vi "Calculate Image MSE.vi"(8 "error in (no error)":errorcluster, 10 "Actual Image":T1, 11 "Expected Image":T1) -> (0 "error out":errorcluster, 3 "MSE":dbl)   [LabVIEW 2020, in "MacroAssert.lvlib" / "Image Assertion.lvclass"]
doc: "Calculates the mean squared error (MSE) between <B>Expected Image</B> and <B>Actual Image</B>."
uses:
  Image Assertion.lvclass
  <vilib>/picture/picture.llb/imagedata.ctl
  <vilib>/Analysis/NI_AALPro.lvlib
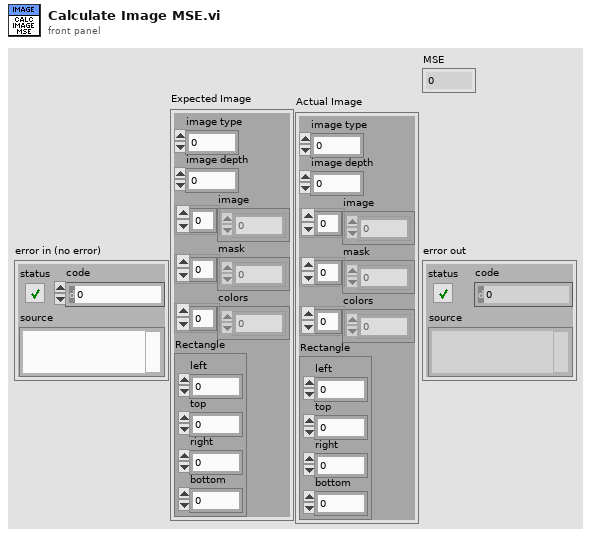
[diagram p1: front panel]
types:
  T1 = typedef "imagedata.ctl" = cluster{"image type":i32, "image depth":i32, "image":u8[], "mask":u8[], "colors":u32[], "Rectangle":cluster{"left":i16, "top":i16, "right":i16, "bottom":i16}}
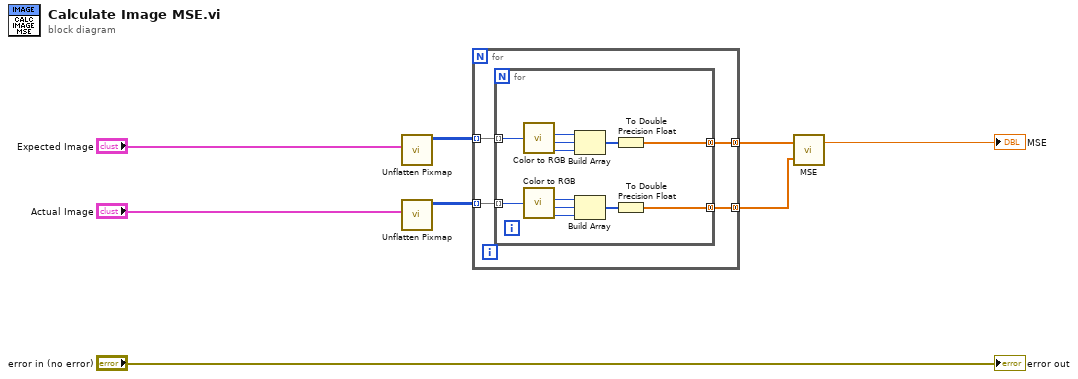
[diagram p0: block diagram]
diagram:
  n1 = call <vilib>:"Unflatten Pixmap.vi"("image data"="Expected Image") -> ("24-bit pixmap"=w4:u32[][])  [unwired: 4 in, 6 out]
  n2 = call <vilib>:"Unflatten Pixmap.vi"("image data"="Actual Image") -> ("24-bit pixmap"=w3:u32[][])  [unwired: 4 in, 6 out]
  n3 = for {
    tunnel: w4 -> [w12] mode=indexing
    tunnel: w3 -> [w11] mode=indexing
    tunnel: [w10] -> w1 mode=concatenating
    tunnel: [w9] -> w2 mode=concatenating
    n4 = for {
      tunnel: w12 -> [w13] mode=indexing
      tunnel: w11 -> [w18] mode=indexing
      tunnel: [w15] -> w10 mode=concatenating
      tunnel: [w14] -> w9 mode=concatenating
      n5 = call <vilib>:"Color to RGB.vi"("Color"=w13) -> ("R"=w24:u8, "G"=w23:u8, "B"=w22:u8)  [unwired: 1 out]
      n6 = call <vilib>:"Color to RGB.vi"("Color"=w18) -> ("R"=w19:u8, "G"=w20:u8, "B"=w21:u8)  [unwired: 1 out]
      n7 = Build Array(w24, w23, w22) -> (w16:u8[])
      n8 = Build Array(w19, w20, w21) -> (w17:u8[])
      n9 = To Double Precision Float(number=w16) -> (double precision float=w15:dbl[])
      n10 = To Double Precision Float(number=w17) -> (double precision float=w14:dbl[])
    }
  }
  n11 = call <vilib>:"MSE.vi"("X Values"=w2, "Y Values"=w1) -> ("mse"=→"MSE":dbl)  [unwired: 1 out]
  "error out" <- "error in (no error)"
